vi "SquareWave (Host).vi"() -> ()   [LabVIEW 2012]
uses:
  <vilib>/FPGAPlugInAG/PCIe-7841R/niLvFpga_Open_PCIe-7841R.vi
  <vilib>/rvi/interface/common/dynamic/niFpgaDynamicAddResources.vi
  <vilib>/Utility/error.llb/Error Cluster From Error Code.vi
  <vilib>/rvi/errors/niLvFpgaAdjustHostInterfaceError.vi
  <vilib>/FPGAPlugInAG/Dynamic/niLvFpga_Close_Dynamic.vi
  <vilib>/rvi/interface/nirviOpenFPGA/nirviOpenFPGA.xnode
  FPGA Bitfiles/OpticsTable_FPGATarget_SquareWave_SmZuxUhsc2E.lvbitx
  <vilib>/rvi/interface/nirviReadWriteControl/nirviReadWriteControl.xnode
  <vilib>/rvi/interface/nirviCloseFPGA/nirviCloseFPGA.xnode
  NiFpgaLv.dll
  <vilib>/rvi/interface/Simulation/niFpgaSimulationCallBeginRW.vi
panel:
  in  "offset":i16(slide) scale=0.0..32000.0
  in  "duty cycle (periods)":dbl(slide)=0.25 scale=0.0..1.0
  in  "amplitude":i16=16000
  in  "frequency (periods/tick)":fxp<+,32,0>=0.0005000000819563866
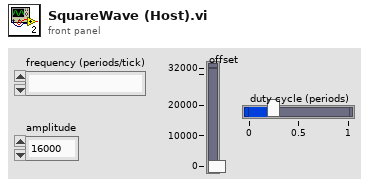
[diagram p1: front panel]
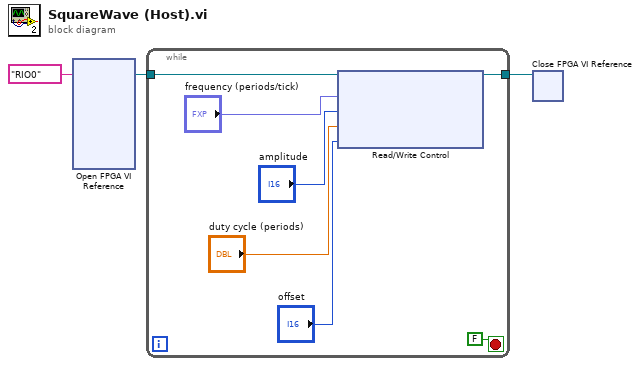
[diagram p0: block diagram]
diagram:
  n1 = xnode "Open FPGA VI Reference"("resource name"=tag "RIO0") -> ("FPGA VI Reference Out"=w2:refnum<k20>)  [unwired: 1 in, 1 out]
  n2 = while {
    tunnel: w2 -> [w10]
    tunnel: [w9] -> w3
    stop <- FALSE stop-if-true
    n3 = xnode "Read/Write Control"("FPGA VI Reference In"=w10, "frequency (periods/tick)"="frequency (periods/tick)", "amplitude"="amplitude", "duty cycle (periods)"="duty cycle (periods)", "offset"="offset") -> ("FPGA VI Reference Out"=w9:refnum<k20>)  [unwired: 1 in, 1 out]
  }
  n4 = xnode "Close FPGA VI Reference"("FPGA VI Reference In"=w3) -> ()  [unwired: 1 in, 1 out]
